vi "GetTestPartValue.vi"(0 "Engine In":refnum<k7>, 5 "SequenceFile In":refnum<k7>, 11 "error in (no error)":errorcluster) -> (4 "Engine Out":refnum<k7>, 6 "SequenceFile Out":refnum<k7>, 15 "error out":errorcluster)   [LabVIEW 2021, in "Create Sequence.lvlib"]
uses:
  Create Sequence.lvlib
  TypeDef/StepProperties.ctl
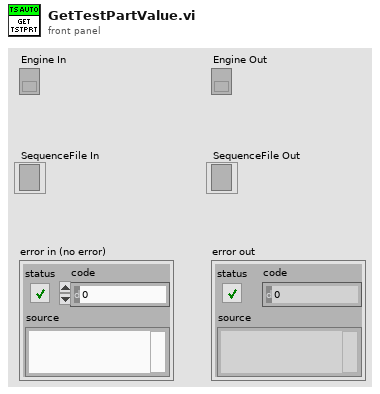
[diagram p1: front panel]
types:
  T1 = typedef "Create Sequence.lvlib/StepProperties.ctl" = cluster{"StepTypeName":string, "StepName":string, "Description":string, "Comment":string, "sequenceNameParam":string, "Step Group":i32, "Step Index":i32, "Expression":string}
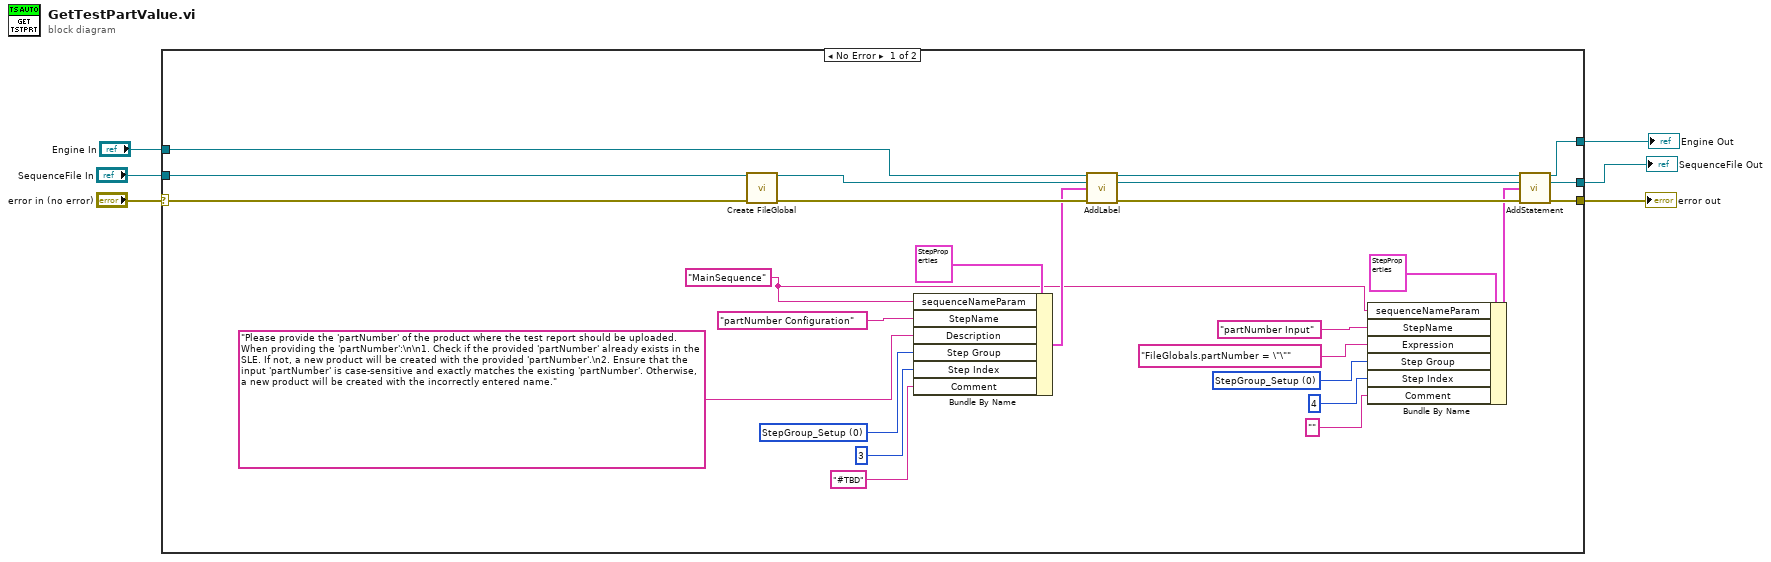
[diagram p0: block diagram]
diagram:
  n1 = case shown="No Error" "error in (no error)" {
    selector: "error in (no error)" -> [w31 w33]
    tunnel: "SequenceFile In" -> [w32 _]
    tunnel: [w30 w33] -> w4
    tunnel: [w29 _] -> w3
    tunnel: [w28 _] -> w2
    tunnel: "Engine In" -> [w20 _]
    frame No Error {
      w7 = "MainSequence" ("sequenceNameParam")
      w11 = 0 items=["StepGroup_Setup", "StepGroup_Main", "StepGroup_Cleanup"] ("Step Group")
      w25 = 0 items=["StepGroup_Setup", "StepGroup_Main", "StepGroup_Cleanup"] ("Step Group")
      n2 = call "Create FileGlobal.vi"("SequenceFile In"=w32, "error in (no error)"=w31) -> ("SequenceFile Out"=w21:refnum<k7>, "error out"=w17:errorcluster)  [unwired: 12 in]
      n3 = Bundle By Name(cluster=T1 {"StepTypeName"="", "StepName"="", "Description"="", "Comment"="", "sequenceNameParam"="MainSequence", "Step Group"=0, "Step Index"=3, "Expression"=""} ("StepProperties"), "sequenceNameParam"=w7, "StepName"="partNumber Configuration" ("Step Name"), "Description"="Please provide the 'partNumber' of the product where the test report should be uploaded. When providing the 'partNumber':\n\n1. Check if the provided 'partNumber' already exists in the SLE. If not, a new product will be created with the provided 'partNumber'.\n2. Ensure that the input 'partNumber' is case-sensitive and exactly matches the existing 'partNumber'. Otherwise, a new product will be created with the incorrectly entered name.", "Step Group"=w25, "Step Index"=3, "Comment"="#TBD") -> (w15:T1)
      n4 = call "AddLabel.vi"("Engine In"=w20, "SequenceFile In"=w21, "StepProperties"=w15, "Error In"=w17) -> ("Engine Out"=w18:refnum<k7>, "SequenceFile Out"=w19:refnum<k7>, "Error Out"=w16:errorcluster)  [unwired: 9 in]
      n5 = Bundle By Name(cluster=T1 {"StepTypeName"="", "StepName"="", "Description"="", "Comment"="", "sequenceNameParam"="MainSequence", "Step Group"=0, "Step Index"=3, "Expression"=""} ("StepProperties"), "sequenceNameParam"=w7, "StepName"="partNumber Input" ("Step Name"), "Expression"="FileGlobals.partNumber = \"\"" ("Description"), "Step Group"=w11, "Step Index"=4, "Comment"="") -> (w8:T1)
      n6 = call "AddStatement.vi"("Engine In"=w18, "SequenceFile In"=w19, "StepProperties"=w8, "Error In"=w16) -> ("Engine Out"=w28:refnum<k7>, "SequenceFile Out"=w29:refnum<k7>, "Error Out"=w30:errorcluster)  [unwired: 9 in]
    }
    frame Error {
    }
  }
  "SequenceFile Out" <- w3
  "error out" <- w4
  "Engine Out" <- w2
